vi "App.Open.vi"(8 "error in (no error)":errorcluster, 11 "State Variables":T1={"Aliases.All"=[], "Aliases.Outputs"=[], "UI.Sequence#ofColumns"=0, "SysDef.Path"=path "", "UI.SequenceRef"=refnum, "UI.StepInformationRef"=refnum, "UI.AbortRef"=refnum, "UI.GraphRef"=refnum, "UI.ViewRef"=refnum, "UI.IterationsRef"=refnum, "UI.IterationInformationRef"=refnum, "INI.Settings"={"Build Location"=path "C:/Simple Sequence Editor/SequenceRepo", "LoggingLocation"=path ""}, "NIVS.Workspace Event"=refnum, "UI.SkipChannel"=refnum, "NIVS.Launched?"=FALSE, "UI.DurationChannel"=refnum}) -> (0 "error out":errorcluster, 3 "State Variables out":T1={"Aliases.All"=[], "Aliases.Outputs"=[], "UI.Sequence#ofColumns"=0, "SysDef.Path"=path "", "UI.SequenceRef"=refnum, "UI.StepInformationRef"=refnum, "UI.AbortRef"=refnum, "UI.GraphRef"=refnum, "UI.ViewRef"=refnum, "UI.IterationsRef"=refnum, "UI.IterationInformationRef"=refnum, "INI.Settings"={"Build Location"=path "C:/Simple Sequence Editor/SequenceRepo", "LoggingLocation"=path ""}, "NIVS.Workspace Event"=refnum, "UI.SkipChannel"=refnum, "NIVS.Launched?"=FALSE, "UI.DurationChannel"=refnum})   [LabVIEW 2015, in "Simple Sequence Tools - Editor.lvlib"]
uses:
  Simple Sequence Tools - Editor.lvlib
  Types/Main.StateVariables.ctl
  Shared/Types/Channel.Properties.ctl
  Shared/Types/INI.Settings.ctl
  Shared/SubVIs/Main.Constants.vi
  Shared/Simple Sequence Tools - Shared.lvlib
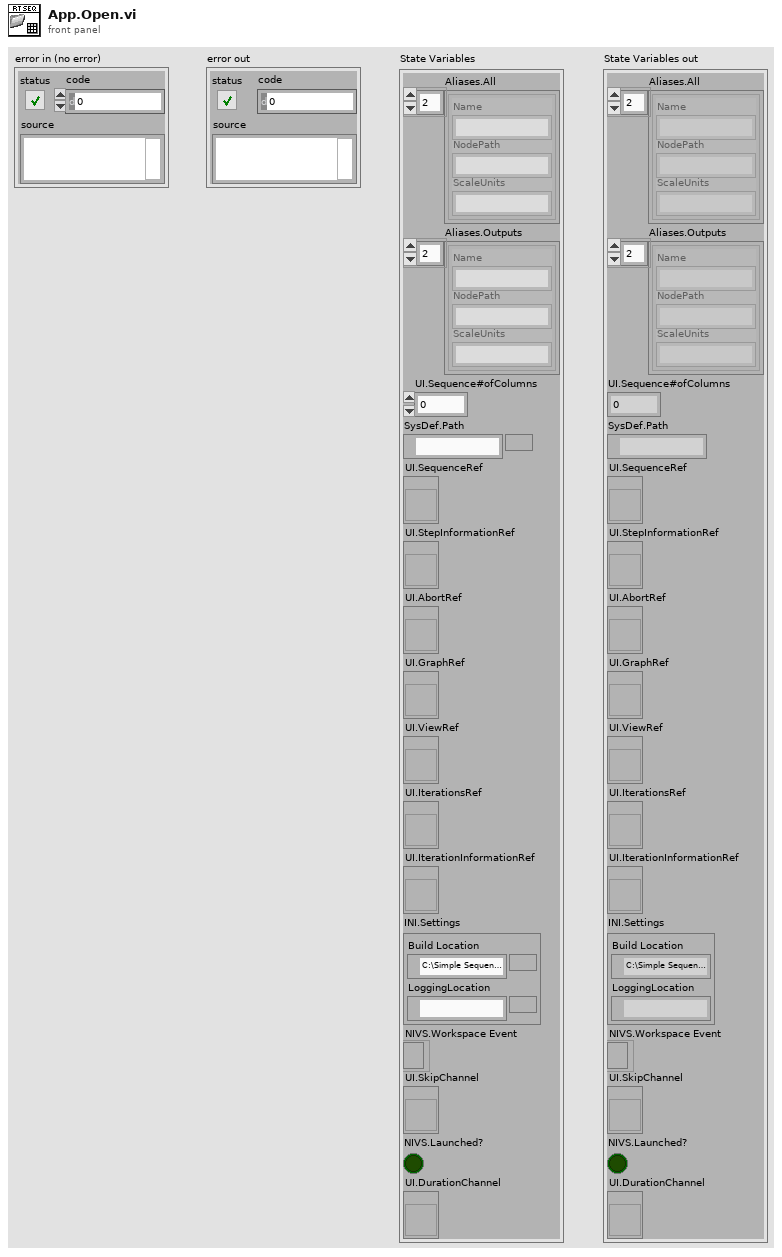
[diagram p1: front panel]
types:
  T1 = typedef "Simple Sequence Tools - Editor.lvlib/Main.StateVariables.ctl" = cluster{"Aliases.All":T2[], "Aliases.Outputs":T2[], "UI.Sequence#ofColumns":i32, "SysDef.Path":path, "UI.SequenceRef":refnum<vi>, "UI.StepInformationRef":refnum<vi>, "UI.AbortRef":refnum<vi>, "UI.GraphRef":refnum<vi>, "UI.ViewRef":refnum<vi>, "UI.IterationsRef":refnum<vi>, "UI.IterationInformationRef":refnum<vi>, "INI.Settings":T3, "NIVS.Workspace Event":refnum<event-registration>, "UI.SkipChannel":refnum<vi>, "NIVS.Launched?":bool, "UI.DurationChannel":refnum<vi>}
  T2 = typedef "Simple Sequence Tools - Shared.lvlib/Channel.Properties.ctl" = cluster{"Name":string, "NodePath":string, "ScaleUnits":string}
  T3 = typedef "Simple Sequence Tools - Shared.lvlib/INI.Settings.ctl" = cluster{"Build Location":path, "LoggingLocation":path}
  T4 = typedef "LVBoundsTypeDef.ctl" = cluster{"Width":u32, "Height":u32}
  T5 = typedef "Simple Sequence Tools - Shared.lvlib/Saved.Sequence.ctl" = cluster{"Output Channels":T2[], "Item Names":string[][], "Step":T2, "Abort":T2, "Iterations":u32, "Iteration":T2, "Skip":T2, "Duration":T2}
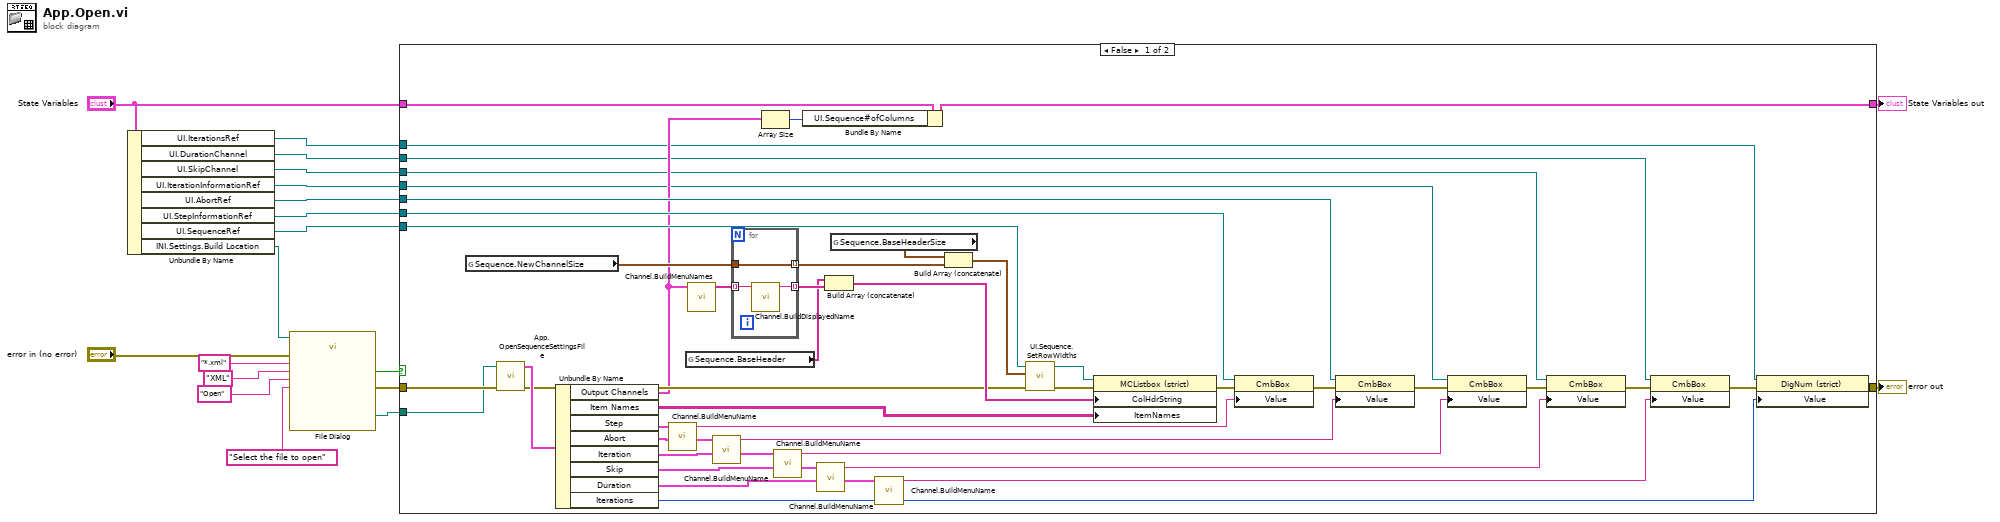
[diagram p0: block diagram]
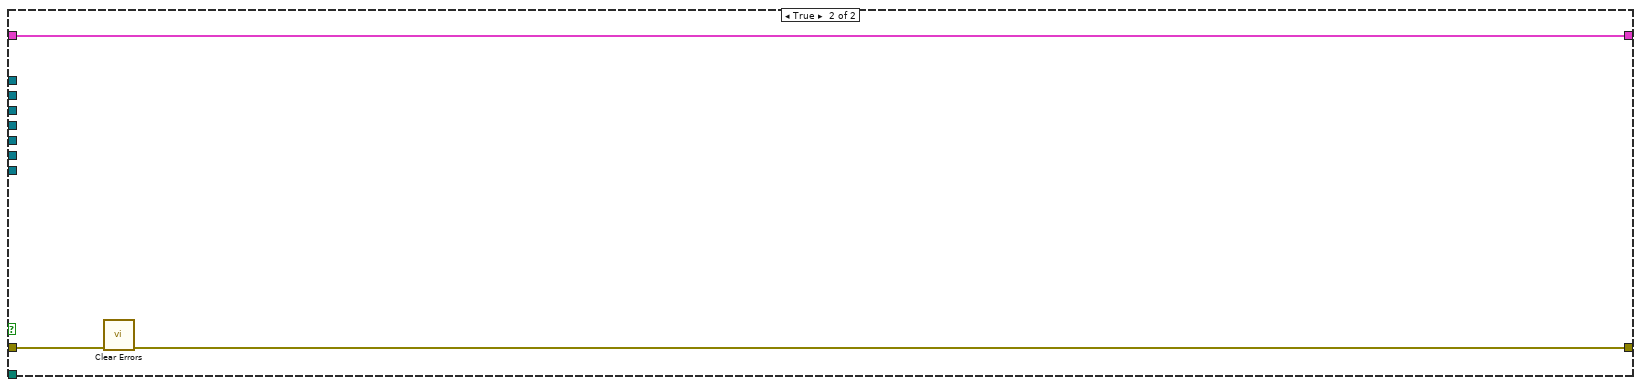
[diagram p2: hidden frame]
diagram:
  n1 = Unbundle By Name("State Variables") -> ("UI.IterationsRef"=w6:refnum<vi>, "UI.DurationChannel"=w1:refnum<vi>, "UI.SkipChannel"=w2:refnum<vi>, "UI.IterationInformationRef"=w5:refnum<vi>, "UI.AbortRef"=w19:refnum<vi>, "UI.StepInformationRef"=w18:refnum<vi>, "UI.SequenceRef"=w17:refnum<vi>, "INI.Settings.Build Location"=w4:path)
  n2 = call "File Dialog"("start path"=w4, "prompt"="Select the file to open", "button label"="Open", "error in"="error in (no error)", "pattern (all files)"="*.xml", "pattern label"="XML") -> ("selected path"=w13:path, "cancelled"=w14:bool, "error out"=w9:errorcluster)  [unwired: 6 in, 1 out]
  n3 = case shown="False" w14 {
    tunnel: [w38 w68] -> w16
    tunnel: w9 -> [w63 w69]
    tunnel: w13 -> [w62 _]
    tunnel: w17 -> [w45 _]
    tunnel: w18 -> [w58 _]
    tunnel: w19 -> [w57 _]
    tunnel: "State Variables" -> [w43 w67]
    tunnel: [w40 w67] -> w7
    tunnel: w6 -> [w39 _]
    tunnel: w5 -> [w35 _]
    tunnel: w2 -> [w33 _]
    tunnel: w1 -> [w30 _]
    frame False {
      n4 = global read "Main.Constants.vi" "Sequence.NewChannelSize"() -> (w52:T4)
      n5 = call "App.OpenSequenceSettingsFile.vi"("error in (no error)"=w63, "selected path"=w62) -> ("error out"=w47:errorcluster, "Settings"=w61:T5)  [unwired: 8 in]
      n6 = Unbundle By Name(w61) -> ("Output Channels"=w42:T2[], "Item Names"=w60:string[][], "Step"=w29:T2, "Abort"=w27:T2, "Iteration"=w25:T2, "Skip"=w23:T2, "Duration"=w21:T2, "Iterations"=w37:u32)
      n7 = call "Channel.BuildMenuName.vi"("cluster"=w29) -> ("NodePath"=w28:string)  [unwired: 10 in]
      n8 = global read "Main.Constants.vi" "Sequence.BaseHeader"() -> (w53:string[])
      n9 = call "Channel.BuildMenuNames.vi"("Aliases"=w42) -> ("Aliases Array"=w59:string[])  [unwired: 10 in]
      n10 = call "Channel.BuildMenuName.vi"("cluster"=w27) -> ("NodePath"=w26:string)  [unwired: 10 in]
      n11 = for {
        tunnel: w59 -> [w66] mode=indexing
        tunnel: [w65] -> w54 mode=indexing
        tunnel: [w64] -> w51 mode=indexing
        tunnel: w52 -> [w64]
        n12 = call "Channel.BuildDisplayedName.vi"("Path"=w66) -> ("Formated Path"=w65:string)  [unwired: 10 in]
      }
      n13 = Array Size(array=w42) -> (size(s)=w41:i32)
      n14 = call "Channel.BuildMenuName.vi"("cluster"=w25) -> ("NodePath"=w24:string)  [unwired: 10 in]
      n15 = Bundle By Name(cluster=w43, "UI.Sequence#ofColumns"=w41) -> (w40:T1)
      n16 = call "Channel.BuildMenuName.vi"("cluster"=w23) -> ("NodePath"=w22:string)  [unwired: 10 in]
      n17 = Build Array (concatenate)(w53, w54) -> (w55:string[])
      n18 = global read "Main.Constants.vi" "Sequence.BaseHeaderSize"() -> (w50:T4[])
      n19 = call "Channel.BuildMenuName.vi"("cluster"=w21) -> ("NodePath"=w20:string)  [unwired: 10 in]
      n20 = Build Array (concatenate)(w50, w51) -> (w49:T4[])
      n21 = call "UI.Sequence.SetRowWidths.vi"("error in (no error)"=w47, "CellSize"=w49, "UI.SequenceRef"=w45) -> ("error out"=w46:errorcluster, "UI.SequenceRef"=w44:refnum<vi>)  [unwired: 7 in]
      n22 = property class="MCListbox (strict)"(reference=w44, error in=w46, "ColHdrString"=w55, "ItemNames"=w60) -> (error out=w48:errorcluster)  [unwired: 1 out]
      n23 = property class="CmbBox"(reference=w58, error in=w48, "Value"=w28) -> (error out=w56:errorcluster)  [unwired: 1 out]
      n24 = property class="CmbBox"(reference=w57, error in=w56, "Value"=w26) -> (error out=w36:errorcluster)  [unwired: 1 out]
      n25 = property class="CmbBox"(reference=w35, error in=w36, "Value"=w24) -> (error out=w34:errorcluster)  [unwired: 1 out]
      n26 = property class="CmbBox"(reference=w33, error in=w34, "Value"=w22) -> (error out=w32:errorcluster)  [unwired: 1 out]
      n27 = property class="CmbBox"(reference=w30, error in=w32, "Value"=w20) -> (error out=w31:errorcluster)  [unwired: 1 out]
      n28 = property class="DigNum (strict)"(reference=w39, error in=w31, "Value"=w37) -> (error out=w38:errorcluster)  [unwired: 1 out]
    }
    frame True {
      n29 = call <vilib>:"Clear Errors.vi"("error in (no error)"=w69) -> ("error out"=w68:errorcluster)  [unwired: 5 in, 1 out]
    }
  }
  "error out" <- w16
  "State Variables out" <- w7
